vi "AB_SplitPaths.vi"(10 "base target path":path, 11 "combined path":path) -> (2 "target path":path, 3 "localDestPath":path)   [LabVIEW 2020]
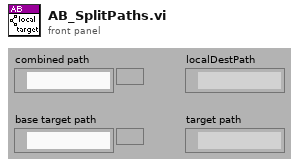
[diagram p1: front panel]
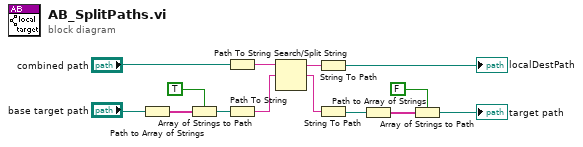
[diagram p0: block diagram]
diagram:
  n1 = Path to Array of Strings(0:"base target path") -> (2:w3:string[])  [unwired: 1 out]
  n2 = Array of Strings to Path(0:w3, 1:TRUE ("relative")) -> (2:w1:path)
  n3 = Path To String(path="combined path") -> (string=w13:string)
  n4 = Path To String(path=w1) -> (string=w12:string)
  n5 = Search/Split String(string=w13, search string/char (-)=w12) -> (substring before match=w11:string, match + rest of string=w9:string)  [unwired: 2 out]
  n6 = String To Path(string=w11) -> (path=→"localDestPath":path)
  n7 = String To Path(string=w9) -> (path=w8:path)
  n8 = Path to Array of Strings(0:w8) -> (2:w7:string[])  [unwired: 1 out]
  n9 = Array of Strings to Path(0:w7, 1:FALSE ("relative")) -> (2:→"target path":path)
